vi "ClearDTCs.vi"(8 "error in (no error)":errorcluster, 9 "timeout ms (1000)":i32=1000, 10 "Group of DTC":u32, 11 "connection info":T1) -> (0 "error out":errorcluster, 3 "connection info":T1)   [LabVIEW 2015, in "Diagnostics Host Automation API.lvlib"]
uses:
  Diagnostics Host Automation API.lvlib
  <vilib>/NI/STM/TCP/TCP Connection Info.ctl
  <vilib>/NI/STM/SubVIs/MetaDataElement.ctl
  <vilib>/NI/NIVS Addon Network Comm/Shared/NI VeriStand Addon Network Comm Shared.lvlib
  <vilib>/NI/STM/NI STM.lvlib
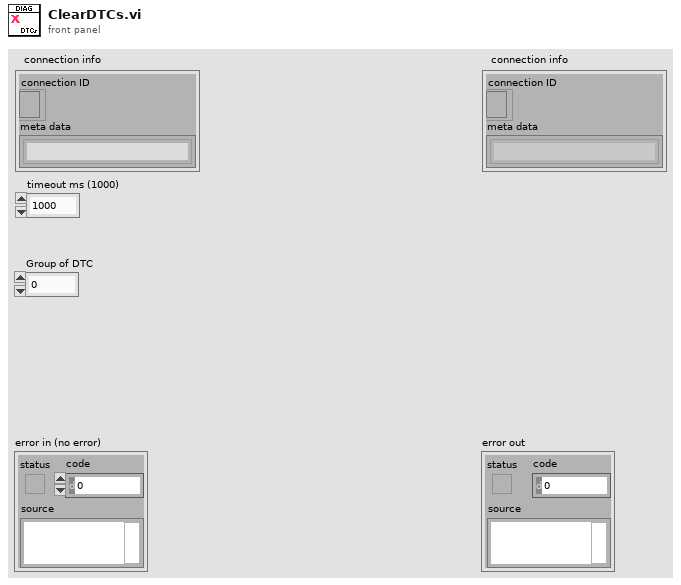
[diagram p1: front panel]
types:
  T1 = typedef "NI STM.lvlib/TCP Connection Info.ctl" = cluster{"connection ID":refnum<k5>, "meta data":T2[]}
  T2 = typedef "NI STM.lvlib/MetaDataElement.ctl" = string
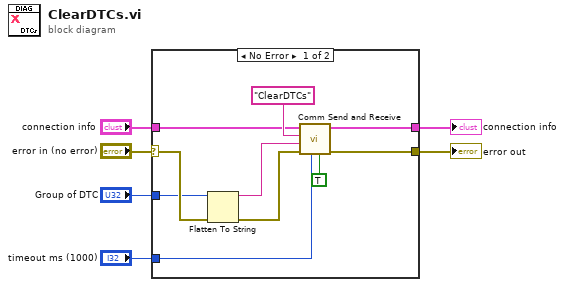
[diagram p0: block diagram]
diagram:
  n1 = case shown="No Error" "error in (no error)" {
    selector: "error in (no error)" -> [w16 w18]
    tunnel: "connection info" -> [w9 w17]
    tunnel: [w8 w17] -> w5
    tunnel: [w10 w18] -> w4
    tunnel: "timeout ms (1000)" -> [w12 _]
    tunnel: "Group of DTC" -> [w15 _]
    frame No Error {
      n2 = Flatten To String(anything=w15, error in (no error)=w16) -> (data string=w13:string, error out=w7:errorcluster)  [unwired: 2 in, 1 out]
      n3 = call <vilib>:"Comm Send and Receive.vi"("Resp Required?"=TRUE, "Timeout (ms)"=w12, "error in (no error)"=w7, "Data"=w13, "Name"="ClearDTCs", "connection info"=w9) -> ("error out"=w10:errorcluster, "connection info"=w8:T1)  [unwired: 2 in, 2 out]
    }
    frame Error {
    }
  }
  "connection info" <- w5
  "error out" <- w4
